vi "Cache_Info Global.vi"() -> ()   [LabVIEW 2020, in "ClassLoader.lvlib"]
uses:
  ClassLoader.lvlib
  Ctl/Ctl_Class Info.ctl
panel:
  in  "Interface Info":map{string, bool}(c390)
  in  "Info":map{string, T1}(c390)
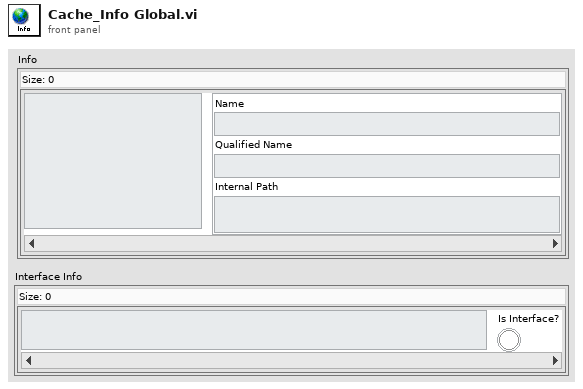
[diagram p1: front panel]
types:
  T1 = typedef "ClassLoader.lvlib/Ctl_Class Info.ctl" = cluster{"Name":string, "Qualified Name":string, "Internal Path":string}
diagram:
